vi "Derivative.vi"() -> ()   [LabVIEW 2023]
panel:
  out "XY Graph 2":cluster{dbl[], dbl[]}(graph)
  out "XY Graph":cluster{dbl[], dbl[]}(graph)
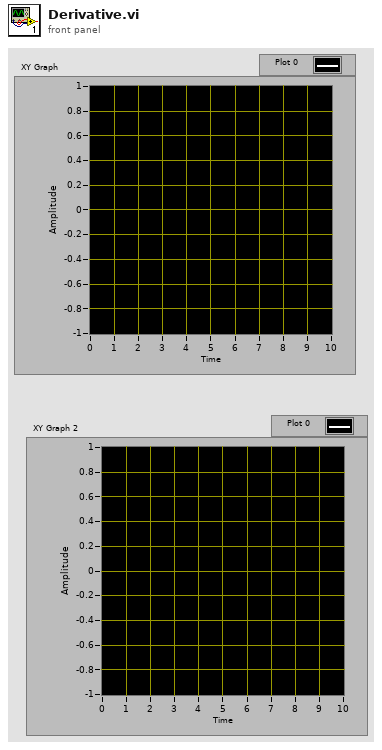
[diagram p1: front panel]
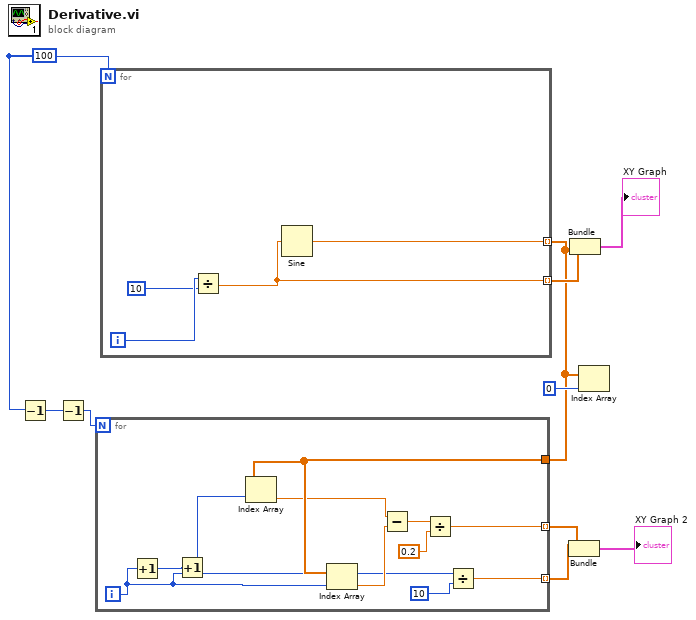
[diagram p0: block diagram]
diagram:
  w7 = 100
  n1 = Decrement(x=w7) -> (x-1=w8:i32)
  n2 = Decrement(x=w8) -> (x-1=w6:i32)
  n3 = for {
    N: w7 -> [_]
    tunnel: [w12] -> w10 mode=indexing
    tunnel: [w11] -> w4 mode=indexing
    i -> [w14]
    n4 = Divide(x=w14, y=10) -> (x/y=w12:dbl)
    n5 = Sine(x=w12) -> (sin(x)=w11:dbl)
  }
  n6 = for {
    N: w6 -> [_]
    tunnel: w4 -> [w23]
    tunnel: [w16] -> w1 mode=indexing
    tunnel: [w15] -> w2 mode=indexing
    i -> [w18]
    n7 = Increment(x=w18) -> (x+1=w25:i32)
    n8 = Increment(x=w25) -> (x+1=w24:i32)
    n9 = Index Array(array=w23, index=w24) -> (element=w22:dbl)
    n10 = Index Array(array=w23, index=w18) -> (element=w21:dbl)
    n11 = Subtract(x=w22, y=w21) -> (x-y=w20:dbl)
    n12 = Divide(x=w20, y=0.2) -> (x/y=w16:dbl)
    n13 = Divide(x=w18, y=10) -> (x/y=w15:dbl)
  }
  n14 = Bundle(w2, w1) -> (→"XY Graph 2":cluster{dbl[], dbl[]})  [unwired: 1 in]
  n15 = Bundle(w10, w4) -> (→"XY Graph":cluster{dbl[], dbl[]})  [unwired: 1 in]
  n16 = Index Array(array=w4, index=0) -> ()  [unwired: 1 out]
